vi "Draw Comparison.vi"(7 "Best Fit":dbl[][](array[numeric]), 10 "Raw Data":dbl[][](array[numeric])) -> (0 "Vertical Comparison":cluster{i32[], dbl[]}[](graph), 3 "Horizontal Comparison":cluster{i32[], dbl[]}[](graph))   [LabVIEW 2013]
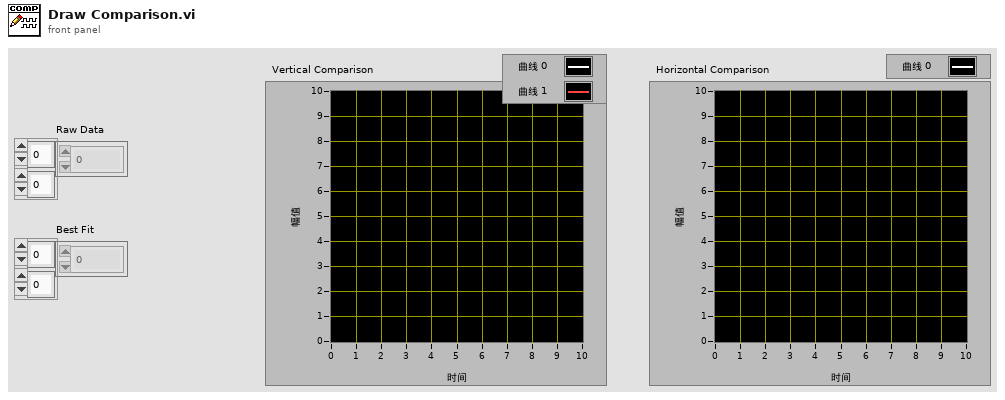
[diagram p1: front panel]
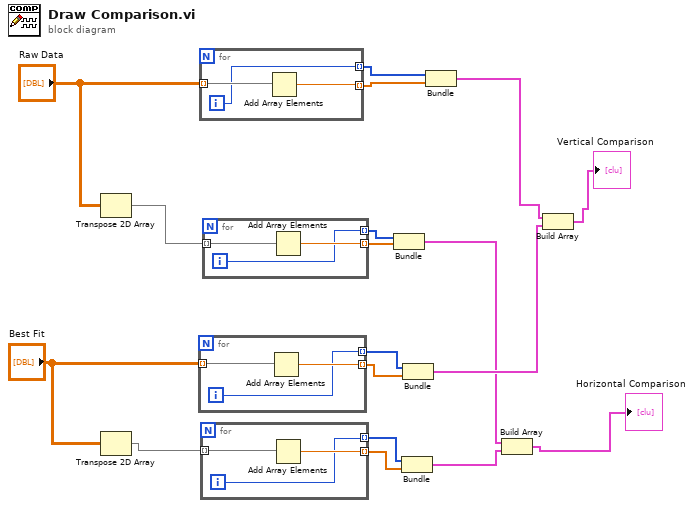
[diagram p0: block diagram]
diagram:
  n1 = Transpose 2D Array(2D array="Raw Data") -> (transposed array=w17:dbl[][])
  n2 = Transpose 2D Array(2D array="Best Fit") -> (transposed array=w15:dbl[][])
  n3 = for {
    tunnel: "Best Fit" -> [w21] mode=indexing
    tunnel: [w20] -> w13 mode=indexing
    tunnel: [w19] -> w9 mode=indexing
    i -> [w19]
    n4 = Add Array Elements(numeric array=w21) -> (sum=w20:dbl)
  }
  n5 = for {
    tunnel: "Raw Data" -> [w24] mode=indexing
    tunnel: [w23] -> w14 mode=indexing
    tunnel: [w22] -> w7 mode=indexing
    i -> [w22]
    n6 = Add Array Elements(numeric array=w24) -> (sum=w23:dbl)
  }
  n7 = for {
    tunnel: w15 -> [w27] mode=indexing
    tunnel: [w26] -> w11 mode=indexing
    tunnel: [w25] -> w10 mode=indexing
    i -> [w25]
    n8 = Add Array Elements(numeric array=w27) -> (sum=w26:dbl)
  }
  n9 = for {
    tunnel: w17 -> [w30] mode=indexing
    tunnel: [w29] -> w12 mode=indexing
    tunnel: [w28] -> w8 mode=indexing
    i -> [w28]
    n10 = Add Array Elements(numeric array=w30) -> (sum=w29:dbl)
  }
  n11 = Bundle(w8, w12) -> (w3:cluster{i32[], dbl[]})  [unwired: 1 in]
  n12 = Bundle(w10, w11) -> (w2:cluster{i32[], dbl[]})  [unwired: 1 in]
  n13 = Bundle(w9, w13) -> (w5:cluster{i32[], dbl[]})  [unwired: 1 in]
  n14 = Bundle(w7, w14) -> (w6:cluster{i32[], dbl[]})  [unwired: 1 in]
  n15 = Build Array(w3, w2) -> (→"Horizontal Comparison":cluster{i32[], dbl[]}[])
  n16 = Build Array(w6, w5) -> (→"Vertical Comparison":cluster{i32[], dbl[]}[])
